vi "Set PCL Decimation.vi"(8 "Error In":errorcluster, 10 "PCL Decimation":u32, 11 "Instrument Addon Refnum In":T1 format="%.0x") -> (0 "Error Out":errorcluster, 3 "Instrument Addon Refnum Out":T1 format="%.0x")   [LabVIEW 2018, in "Instrument Addon Scripting API.lvlib"]
doc: "Returns the PCL Decimation value set for the Instrument Addon Custom Device\n\nInput:\nInstrument Addon Refnum In: represents the refference number to an Instrument Addon Custom Device\nPCL Decimation: value which will be set for PCL Decimation (default is 0)\n\nOutput:\nInstrument Addon Refnum Out: represents the refference number to the Instrument Addon Custom Device provided as an input"
uses:
  Instrument Addon Scripting API.lvlib
  <vilib>/NI Veristand/Custom Device API/Custom Device Item Ref.ctl
  Addon/Addon Shared/SubVIs/Constants.vi
  <vilib>/NI/NI VeriStand Advanced SysDef API/_SubVIs/SysDef.Property.Set.U32.vi
  Addon/Addon Shared/Instrument Addon Shared.lvlib
  <vilib>/NI/NI VeriStand Advanced SysDef API/SysDef API/Advanced System Definition.lvlib
  <vilib>/NI Veristand/Custom Device API/Custom Device API.lvlib
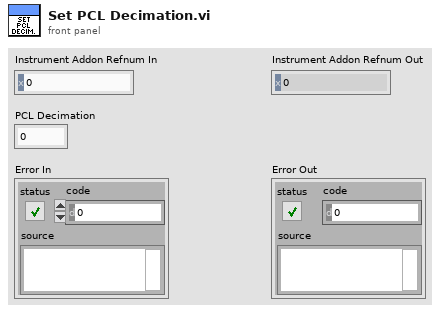
[diagram p1: front panel]
types:
  T1 = typedef "Custom Device API.lvlib/Custom Device Item Ref.ctl" = u64
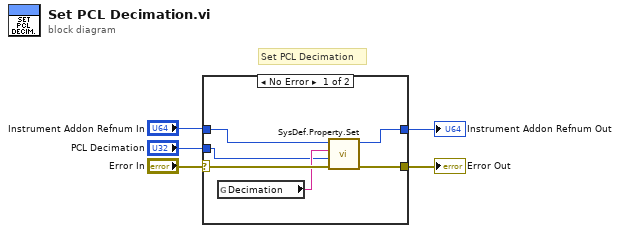
[diagram p0: block diagram]
diagram:
  # "Set PCL Decimation"
  n1 = case shown="No Error" "Error In" {
    selector: "Error In" -> [w11 w13]
    tunnel: "Instrument Addon Refnum In" -> [w8 w12]
    tunnel: [w7 w13] -> w4
    tunnel: [w6 w12] -> w1
    tunnel: "PCL Decimation" -> [w9 _]
    frame No Error {
      n2 = global read "Constants.vi" "Decimation"() -> (w10:string)
      n3 = call-poly <vilib>:"SysDef.Property.Set.vi"("error in (no error)"=w11, "Value"=w9, "Property Name"=w10, "nodeID"=w8) -> ("error out"=w7:errorcluster, "nodeID out"=w6:u64)  [unwired: 6 in]
    }
    frame Error {
    }
  }
  "Error Out" <- w4
  "Instrument Addon Refnum Out" <- w1
